vi "Read Timeout.vi"(8 "Error In":errorcluster) -> (0 "Error Out":errorcluster)   [LabVIEW 2018, in "Tests.lvlib" / "Session.lvlib"]
uses:
  Session.lvlib
  <vilib>/addons/_JKI Toolkits/Caraya/classes/Test/Test.lvclass
  src/Toolkit/SSH/SSH.lvclass
  src/Toolkit/Session/Session.lvclass
  <vilib>/addons/_JKI Toolkits/Caraya/classes/Assert/Assert.lvclass
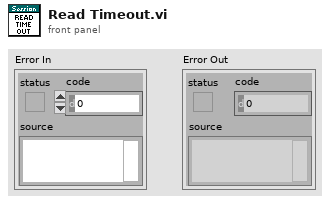
[diagram p1: front panel]
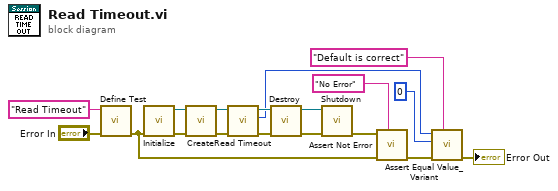
[diagram p0: block diagram]
diagram:
  n1 = call <vilib>:"Define Test.vi"("error in (no error)"="Error In", "Label (VI Title)"="Read Timeout") -> ("error out"=w10:errorcluster)  [unwired: 9 in]
  n2 = call "Initialize.vi"("Error In"=w10) -> ("Error Out"=w16:errorcluster, "SSH"=w15:refnum<class "SSH.lvclass">)  [unwired: 9 in]
  n3 = call "Create.vi"("Error In"=w16, "SSH"=w15) -> ("Error Out"=w5:errorcluster, "Sesssion"=w6:refnum<class "Session.lvclass">)  [unwired: 8 in]
  n4 = call "Read Timeout.vi"("Error In"=w5, "Session In"=w6) -> ("Error Out"=w4:errorcluster, "Timeout"=w2:i32, "Sesssion Out"=w3:refnum<class "Session.lvclass">)  [unwired: 7 in]
  n5 = call "Destroy.vi"("Error In"=w4, "Session"=w3) -> ("Error Out"=w13:errorcluster, "SSH"=w14:refnum<class "SSH.lvclass">)  [unwired: 8 in]
  n6 = call "Shutdown.vi"("Error In"=w13, "SSH"=w14) -> ("Error Out"=w12:errorcluster)  [unwired: 9 in]
  n7 = call <vilib>:"Assert Not Error.vi"("Label"="No Error", "error in (no error)"=w10, "Not Error?"=w12) -> ("error out"=w9:errorcluster)  [unwired: 8 in]
  n8 = call <vilib>:"Assert Equal Value_Variant.vi"("Label"="Default is correct", "error in (no error)"=w9, "Y"=0 ("Timeout"), "X"=w2) -> ("error out"=→"Error Out":errorcluster)  [unwired: 7 in]
